vi "base64 encode.vi"(10 "string in (not encoded)":string) -> (2 "string out (base64-encoded)":string)   [LabVIEW 2016, in "websocket core.lvlib"]
uses:
  websocket core.lvlib
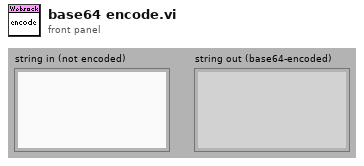
[diagram p1: front panel]
types:
  T1 = cluster{"unsigned byte array[0]":u8, "unsigned byte array[1]":u8, "unsigned byte array[2]":u8}
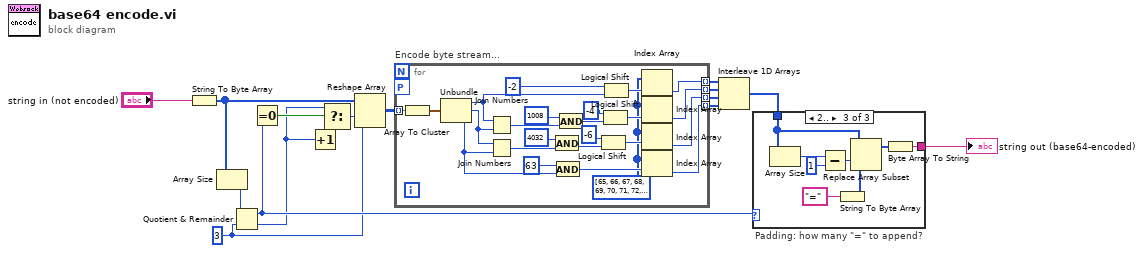
[diagram p0: block diagram]
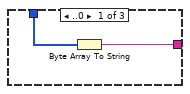
[diagram p2: hidden frame]
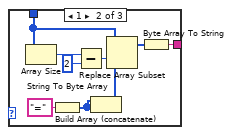
[diagram p3: hidden frame]
diagram:
  w3 = 3 ("y")
  n1 = String To Byte Array(string="string in (not encoded)") -> (unsigned byte array=w4:u8[])
  n2 = Array Size(array=w4) -> (size(s)=w12:i32)
  n3 = Quotient & Remainder(x=w12, y=w3) -> (x-y*floor(x/y)=w13:i32, floor(x/y)=w6:i32)
  n4 = Equal To 0?(x=w13) -> (x = 0?=w14:bool)
  n5 = Increment(x=w6) -> (x+1=w7:i32)
  n6 = Select(t=w6, s=w14, f=w7) -> (s? t:f=w2:i32)
  n7 = Reshape Array(w4, w2, w3) -> (w1:u8[][])
  n8 = for "Encode byte stream..." {
    tunnel: [w19] -> w8 mode=indexing
    tunnel: [w20] -> w9 mode=indexing
    tunnel: [w21] -> w10 mode=indexing
    tunnel: [w22] -> w11 mode=indexing
    workers-P: _ -> [_]
    tunnel: w1 -> [w17] mode=indexing
    w18 = u8[] [65, 66, 67, 68, 69, 70, 71, 72, 73, 74, 75, 76, 77, 78, 79, 80, 81, 82, 83, 84, 85, 86, 87, 88, 89, 90, 97, 98, 99, 100, 101, 102, 103, 104, 105, 106, 107, 108, 109, 110, 111, 112, 113, 114, 115, 116, 117, 118, 119, 120, 121, 122, 48, 49, 50, 51, 52, 53, 54, 55, 56, 57, 43, 47] ("unsigned byte array")
    n9 = Array To Cluster(array=w17) -> (cluster=w40:T1)
    n10 = Unbundle(w40) -> ("unsigned byte array[0]"=w29:u8, "unsigned byte array[1]"=w34:u8, "unsigned byte array[2]"=w28:u8)
    n11 = Join Numbers(hi=w29, lo=w34) -> ((hi.lo)=w38:u16)
    n12 = Join Numbers(hi=w34, lo=w28) -> ((hi.lo)=w33:u16)
    n13 = And(x=u16 4032, y=w33) -> (x .and. y?=w31:u16)
    n14 = And(x=u8 63, y=w28) -> (x .and. y?=w23:u8)
    n15 = And(x=u16 1008, y=w38) -> (x .and. y?=w36:u16)
    n16 = Logical Shift(y=i8 -6, x=w31) -> (x << y=w24:u16)
    n17 = Logical Shift(y=i8 -4, x=w36) -> (x << y=w25:u16)
    n18 = Logical Shift(y=i8 -2, x=w29) -> (x << y=w26:u8)
    n19 = Index Array(array=w18, index=w26) -> (element=w22:u8)
    n20 = Index Array(array=w18, index=w25) -> (element=w21:u8)
    n21 = Index Array(array=w18, index=w24) -> (element=w20:u8)
    n22 = Index Array(array=w18, index=w23) -> (element=w19:u8)
  }
  n23 = Interleave 1D Arrays(w11, w10, w9, w8) -> (w5:u8[])
  n24 = case "Padding: how many \"=\" to append?" shown="2.." w13 {
    tunnel: [w41 w48 w56] -> w15
    tunnel: w5 -> [w42 w46 w54]
    frame ..0 {
      n25 = Byte Array To String(unsigned byte array=w42) -> (string=w41:string)
    }
    frame 1 {
      n26 = Array Size(array=w46) -> (size(s)=w47:i32)
      n27 = String To Byte Array(string="=") -> (unsigned byte array=w44:u8[])
      n28 = Subtract(x=w47, y=2) -> (x-y=w50:i32)
      n29 = Build Array (concatenate)(w44, w44) -> (w43:u8[])
      n30 = Replace Array Subset(array=w46, new element=w43, index=w50) -> (w49:u8[])
      n31 = Byte Array To String(unsigned byte array=w49) -> (string=w48:string)
    }
    frame 2.. {
      n32 = Array Size(array=w54) -> (size(s)=w55:i32)
      n33 = Subtract(x=w55, y=1) -> (x-y=w58:i32)
      n34 = String To Byte Array(string="=") -> (unsigned byte array=w52:u8[])
      n35 = Replace Array Subset(array=w54, new element=w52, index=w58) -> (w57:u8[])
      n36 = Byte Array To String(unsigned byte array=w57) -> (string=w56:string)
    }
  }
  "string out (base64-encoded)" <- w15
